vi "Monitor_set.vi"(8 "error in":errorcluster, 11 "Tab Control":refnum<vi>) -> (0 "error out":errorcluster)   [LabVIEW 2015]
uses:
  Global/Globalclient.vi
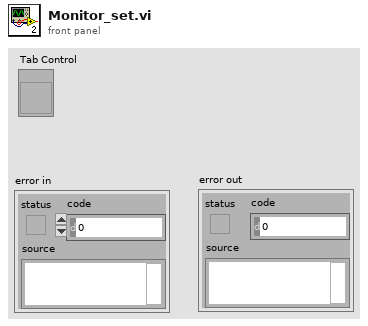
[diagram p1: front panel]
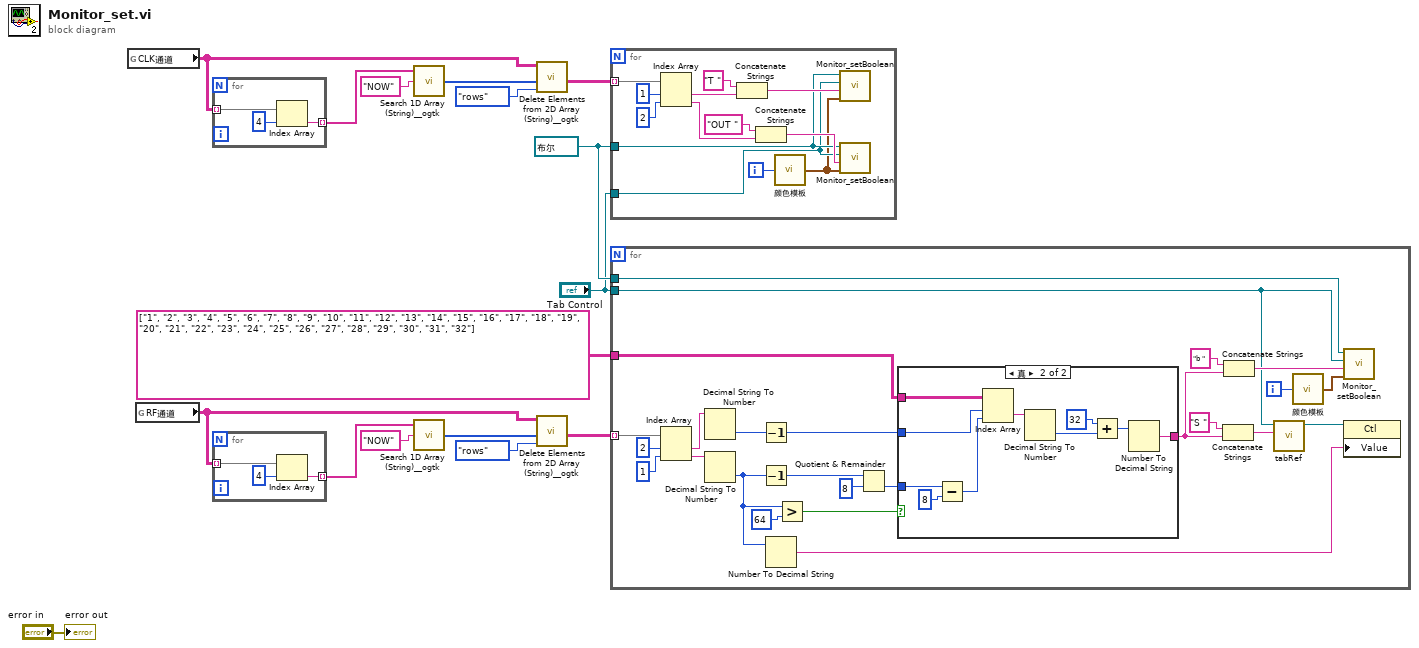
[diagram p0: block diagram]
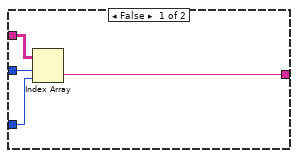
[diagram p2: hidden frame]
diagram:
  w2 = refnum<vi> refnum ("dup reference")
  n1 = global read "Globalclient.vi" "CLK通道"() -> (w5:string[][])
  n2 = global read "Globalclient.vi" "RF通道"() -> (w6:string[][])
  n3 = for {
    tunnel: w5 -> [w19] mode=indexing
    tunnel: [w17] -> w10 mode=indexing
    n4 = Index Array(array=w19, index=4) -> (element=w17:string)
  }
  n5 = for {
    tunnel: w6 -> [w22] mode=indexing
    tunnel: [w20] -> w13 mode=indexing
    n6 = Index Array(array=w22, index=4) -> (element=w20:string)
  }
  n7 = call <userlib>:"Search 1D Array (String)__ogtk.vi"("Array"=w10, "Element Data"="NOW") -> ("Indices of Elements"=w9:i32[])  [unwired: 7 in]
  n8 = call <userlib>:"Search 1D Array (String)__ogtk.vi"("Array"=w13, "Element Data"="NOW") -> ("Indices of Elements"=w14:i32[])  [unwired: 7 in]
  n9 = call <userlib>:"Delete Elements from 2D Array (String)__ogtk.vi"("delete (rows or columns)"=enum16{"rows", "columns"}."rows", "indices"=w9, "array"=w5) -> ("deleted elements"=w3:string[][])  [unwired: 7 in, 1 out]
  n10 = call <userlib>:"Delete Elements from 2D Array (String)__ogtk.vi"("delete (rows or columns)"=enum16{"rows", "columns"}."rows", "indices"=w14, "array"=w6) -> ("deleted elements"=w4:string[][])  [unwired: 7 in, 1 out]
  n11 = for {
    tunnel: w3 -> [w27] mode=indexing
    tunnel: w2 -> [w26]
    tunnel: "Tab Control" -> [w25]
    i -> [w24]
    n12 = Index Array(array=w27, index #1=1 ("index"), index #2=2 ("index")) -> (element #1=w34:string, element #2=w35:string)
    n13 = Concatenate Strings("T " ("format string"), w34) -> (w30:string)
    n14 = Concatenate Strings("OUT " ("format string"), w35) -> (w31:string)
    n15 = call "颜色模板.vi"("Color"=w24) -> ("ColorModule"=w23:cluster{u32, u32}[])
    n16 = call "Monitor_setBoolean.vi"("ColorModule"=w23, "ControlName"=w30, "Tab Control"=w25, "Boolean in"=w26) -> ()
    n17 = call "Monitor_setBoolean.vi"("ColorModule"=w23, "ControlName"=w31, "Tab Control"=w25, "Boolean in"=w26) -> ()
  }
  n18 = for {
    tunnel: string[][] [["1", "2", "3", "4", "5", "6", "7", "8"], ["9", "10", "11", "12", "13", "14", "15", "16"], ["17", "18", "19", "20", "21", "22", "23", "24"], ["25", "26", "27", "28", "29", "30", "31", "32"]] -> [w50]
    tunnel: w4 -> [w46] mode=indexing
    tunnel: w2 -> [w39]
    tunnel: "Tab Control" -> [w36]
    i -> [w38]
    n19 = Index Array(array=w46, index #1=2 ("index"), index #2=1 ("index")) -> (element #1=w43:string, element #2=w41:string)
    n20 = Decimal String To Number(string=w43) -> (number=w42:i32)  [unwired: 2 in, 1 out]
    n21 = Decimal String To Number(string=w41) -> (number=w40:i32)  [unwired: 2 in, 1 out]
    n22 = Decrement(x=w42) -> (x-1=w48:i32)
    n23 = Decrement(x=w40) -> (x-1=w59:i32)
    n24 = Number To Decimal String(number=w40) -> (decimal integer string=w56:string)  [unwired: 1 in]
    n25 = Greater?(x=w40, y=64) -> (0:w51:bool)
    n26 = Quotient & Remainder(x=w59, y=8) -> (floor(x/y)=w47:i32)  [unwired: 1 out]
    n27 = case shown="真" w51 {
      tunnel: w50 -> [w64 w73]
      tunnel: [w63 w65] -> w49
      tunnel: w48 -> [w62 w74]
      tunnel: w47 -> [w61 w72]
      frame False {
        n28 = Index Array(array=w64, index (row)=w62, index (col)=w61) -> (element=w63:string)
      }
      frame True {
        n29 = Subtract(x=w72, y=8) -> (x-y=w70:i32)
        n30 = Index Array(array=w73, index (row)=w74, index (col)=w70) -> (element=w69:string)
        n31 = Decimal String To Number(string=w69) -> (number=w68:i32)  [unwired: 2 in, 1 out]
        n32 = Add(x=32, y=w68) -> (x+y=w66:i32)
        n33 = Number To Decimal String(number=w66) -> (decimal integer string=w65:string)  [unwired: 1 in]
      }
    }
    n34 = Concatenate Strings("S " ("format string"), w49) -> (w54:string)
    n35 = Concatenate Strings("b ", w49) -> (w53:string)
    n36 = call "tabRef.vi"("control name"=w54, "Tab Control"=w36) -> ("control refnum"=w57:refnum<vi>)  [unwired: 8 in, 1 out]
    n37 = call "颜色模板.vi"("Color"=w38) -> ("ColorModule"=w37:cluster{u32, u32}[])
    n38 = call "Monitor_setBoolean.vi"("ColorModule"=w37, "ControlName"=w53, "Tab Control"=w36, "Boolean in"=w39) -> ()
    n39 = property class="Ctl"(reference=w57, "Value"=w56) -> ()  [unwired: 1 in, 2 out]
  }
  "error out" <- "error in"
